vi "load_I_T_from_file.vi"() -> ()   [LabVIEW 2016]
uses:
  <vilib>/Utility/file.llb/Read Delimited Spreadsheet (DBL).vi
panel:
  out "Inputs Shuffled":dbl[][](array[numeric])
  out "Targets Shuffled":dbl[][](array[numeric])
  in  "Proceed to Input Data":bool
  in  "# Nodes Per Stage":dbl[](array[numeric])
  in  "# Hidden Layers":dbl
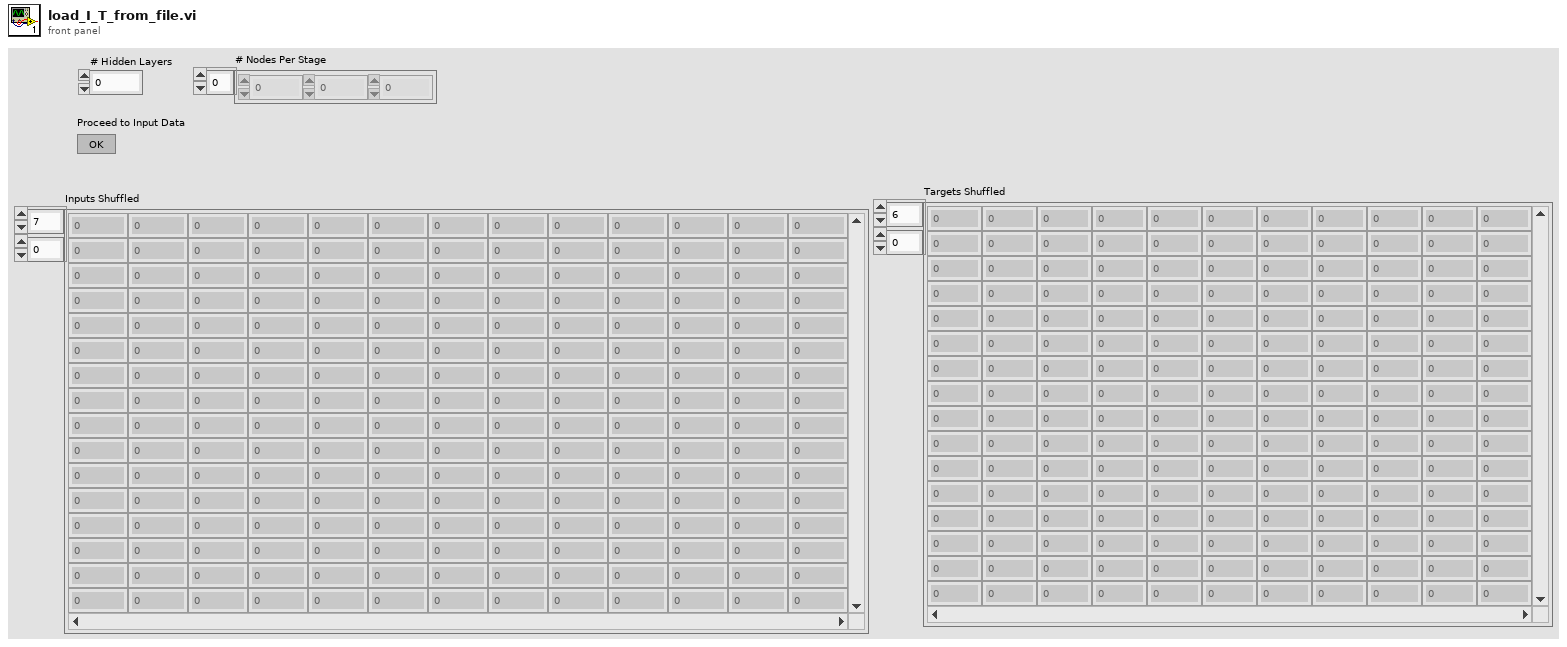
[diagram p1: front panel]
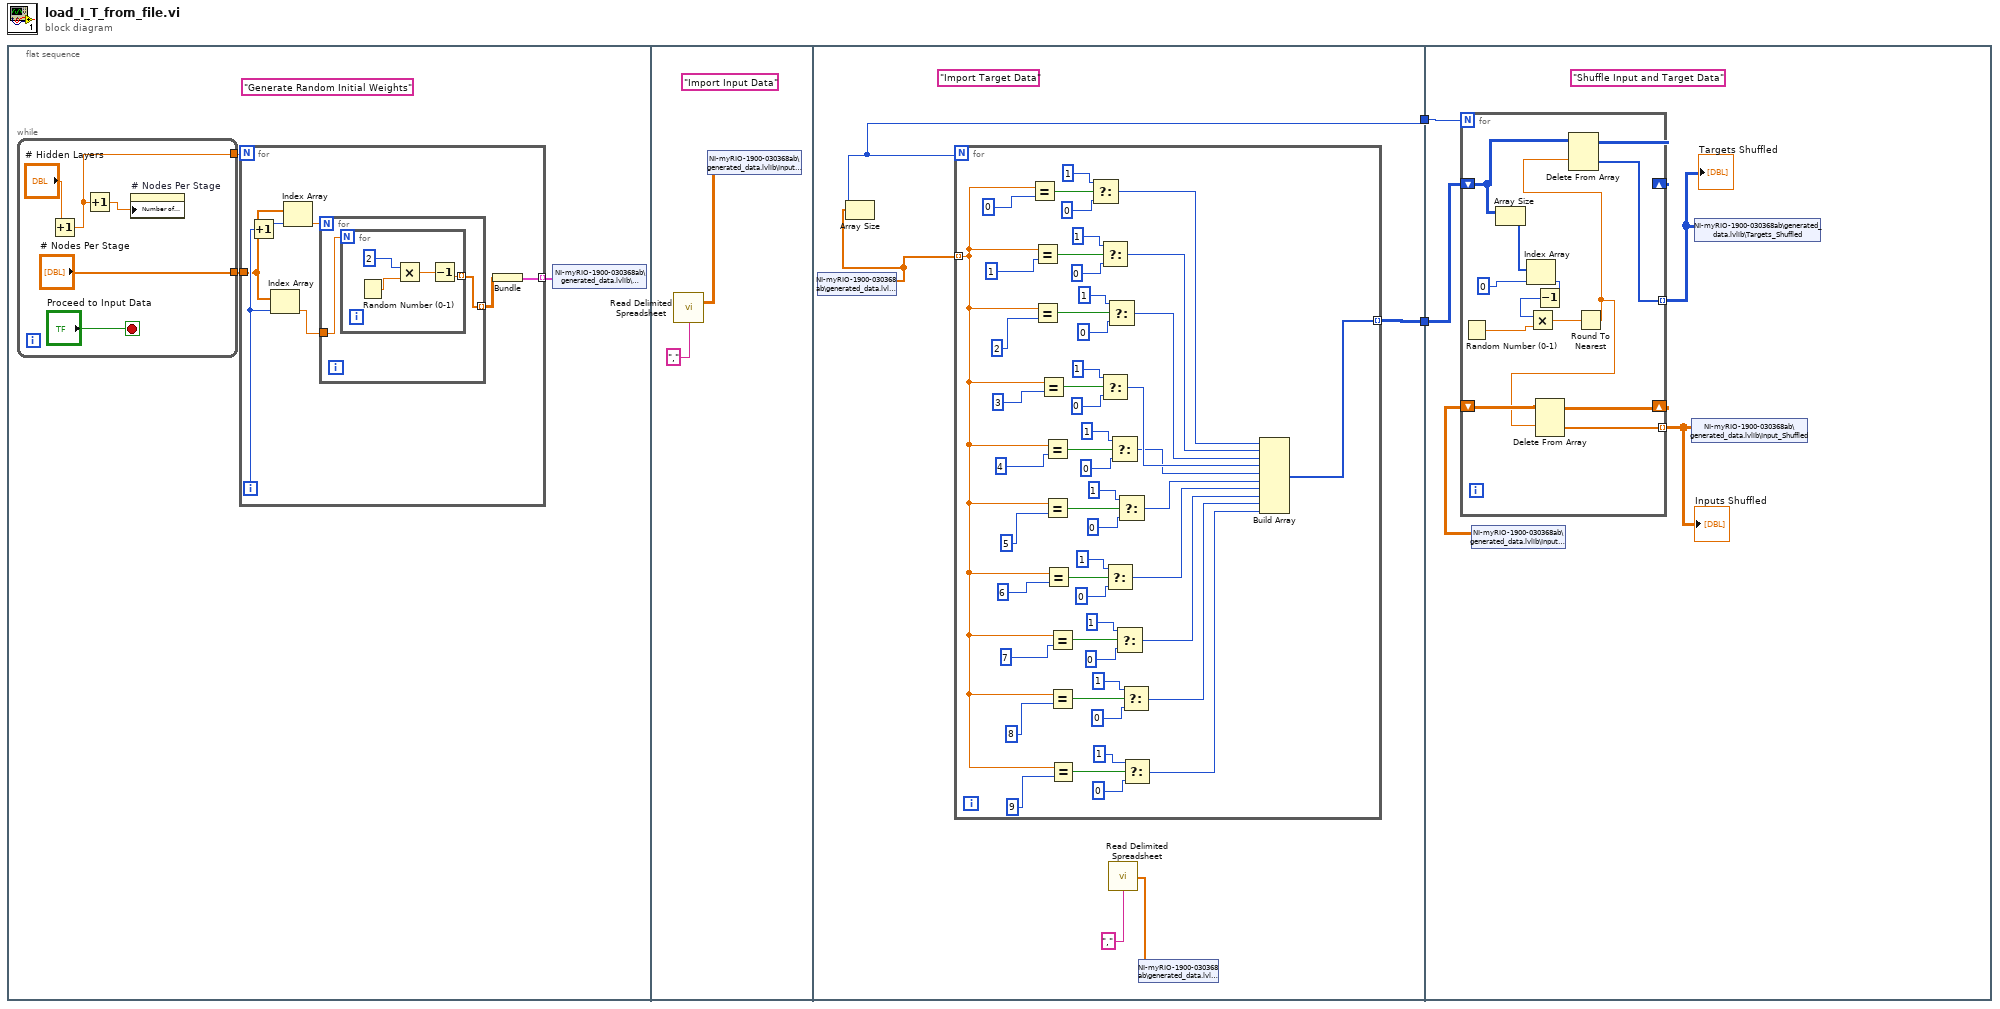
[diagram p0: block diagram]
diagram:
  n1 = flat-sequence {
    tunnel: [w28] -> w2
    tunnel: [w27] -> w1
    tunnel: w2 -> [w87]
    tunnel: w1 -> [w83]
    frame #0 {
      (unwired) "Generate Random Initial Weights"
      n2 = while {
        tunnel: [w8] -> w4
        tunnel: ["# Nodes Per Stage"] -> w3
        stop <- "Proceed to Input Data" stop-if-true
        n3 = Increment(x="# Hidden Layers") -> (x+1=w8:dbl)
        n4 = Increment(x=w8) -> (x+1=w6:dbl)
        n5 = property on="# Nodes Per Stage" class="Arr (strict)"("Number of Columns"=w6) -> ()  [unwired: 2 in, 2 out]
      }
      n6 = for {
        N: w4 -> [_]
        tunnel: [w17] -> w5 mode=indexing
        tunnel: w3 -> [w14]
        i -> [w16]
        n7 = Increment(x=w16) -> (x+1=w15:i32)
        n8 = Index Array(array=w14, index=w16) -> (element=w12:dbl)
        n9 = Index Array(array=w14, index=w15) -> (element=w13:dbl)
        n10 = for {
          N: w13 -> [_]
          tunnel: [w19] -> w11 mode=indexing
          tunnel: w12 -> [w18]
          n11 = for {
            N: w18 -> [_]
            tunnel: [w23] -> w19 mode=indexing
            n12 = Random Number (0-1)() -> (number: 0 to 1=w21:dbl)
            n13 = Multiply(x=2, y=w21) -> (x*y=w20:dbl)
            n14 = Decrement(x=w20) -> (x-1=w23:dbl)
          }
        }
        n15 = Bundle(w11) -> (w17:cluster{dbl[][]})  [unwired: 1 in]
      }
      n16 = shared-variable "NI-myRIO-1900-030368ab\\generated_data.lvlib\\Weights_1"(w5) -> ()  [unwired: 1 in, 1 out]
    }
    frame #1 {
      (unwired) "Import Input Data"
      n17 = call-poly <vilib>:"Read Delimited Spreadsheet.vi"("delimiter (\\t)"=",") -> ("all rows"=w24:dbl[][])  [unwired: 9 in, 5 out]
      n18 = shared-variable "NI-myRIO-1900-030368ab\\generated_data.lvlib\\Input Data"(w24) -> ()  [unwired: 1 in, 1 out]
    }
    frame #2 {
      (unwired) "Import Target Data"
      n19 = shared-variable "NI-myRIO-1900-030368ab\\generated_data.lvlib\\Targets"() -> (w26:dbl[])  [unwired: 1 in, 1 out]
      n20 = Array Size(array=w26) -> (size(s)=w27:i32)
      n21 = for {
        N: w27 -> [_]
        tunnel: w26 -> [w39] mode=indexing
        tunnel: [w67] -> w28 mode=indexing
        n22 = Equal?(x=w39, y=0) -> (x = y?=w79:bool)
        n23 = Equal?(x=w39, y=1) -> (x = y?=w71:bool)
        n24 = Equal?(x=w39, y=2) -> (x = y?=w72:bool)
        n25 = Equal?(x=w39, y=3) -> (x = y?=w63:bool)
        n26 = Equal?(x=w39, y=4) -> (x = y?=w55:bool)
        n27 = Equal?(x=w39, y=5) -> (x = y?=w56:bool)
        n28 = Equal?(x=w39, y=6) -> (x = y?=w51:bool)
        n29 = Equal?(x=w39, y=7) -> (x = y?=w43:bool)
        n30 = Equal?(x=w39, y=8) -> (x = y?=w44:bool)
        n31 = Equal?(x=w39, y=9) -> (x = y?=w40:bool)
        n32 = Select(t=1, s=w79, f=0) -> (s? t:f=w70:i32)
        n33 = Select(t=1, s=w71, f=0) -> (s? t:f=w69:i32)
        n34 = Select(t=1, s=w63, f=0) -> (s? t:f=w38:i32)
        n35 = Select(t=1, s=w51, f=0) -> (s? t:f=w35:i32)
        n36 = Select(t=1, s=w72, f=0) -> (s? t:f=w68:i32)
        n37 = Select(t=1, s=w55, f=0) -> (s? t:f=w37:i32)
        n38 = Select(t=1, s=w43, f=0) -> (s? t:f=w34:i32)
        n39 = Select(t=1, s=w56, f=0) -> (s? t:f=w36:i32)
        n40 = Select(t=1, s=w44, f=0) -> (s? t:f=w33:i32)
        n41 = Select(t=1, s=w40, f=0) -> (s? t:f=w32:i32)
        n42 = Build Array(w70, w69, w68, w38, w37, w36, w35, w34, w33, w32) -> (w67:i32[])
      }
      n43 = call-poly <vilib>:"Read Delimited Spreadsheet.vi"("delimiter (\\t)"=",") -> ("first row"=w30:dbl[])  [unwired: 9 in, 5 out]
      n44 = shared-variable "NI-myRIO-1900-030368ab\\generated_data.lvlib\\Targets"(w30) -> ()  [unwired: 1 in, 1 out]
    }
    frame #3 {
      (unwired) "Shuffle Input and Target Data"
      n45 = shared-variable "NI-myRIO-1900-030368ab\\generated_data.lvlib\\Input Data"() -> (w84:dbl[][])  [unwired: 1 in, 1 out]
      n46 = for {
        N: w83 -> [_]
        shift-right: [w100] -> _
        shift-left: w87 -> [w99]
        tunnel: [w90] -> w86 mode=indexing
        shift-right: [w92] -> _
        shift-left: w84 -> [w93]
        tunnel: [w89] -> w85 mode=indexing
        n47 = Random Number (0-1)() -> (number: 0 to 1=w98:dbl)
        n48 = Array Size(array=w99) -> (size(s)=w96:i32[])
        n49 = Index Array(array=w96, index=0) -> (element=w95:i32)
        n50 = Decrement(x=w95) -> (x-1=w88:i32)
        n51 = Multiply(x=w88, y=w98) -> (x*y=w97:dbl)
        n52 = Round To Nearest(number=w97) -> (nearest integer value=w91:dbl)
        n53 = Delete From Array(array=w93, index (row)=w91) -> (deleted portion=w89:dbl[], array with subset deleted=w92:dbl[][])  [unwired: 2 in]
        n54 = Delete From Array(array=w99, index (row)=w91) -> (deleted portion=w90:i32[], array with subset deleted=w100:i32[][])  [unwired: 2 in]
      }
      "Targets Shuffled" <- w86
      "Inputs Shuffled" <- w85
      n55 = shared-variable "NI-myRIO-1900-030368ab\\generated_data.lvlib\\Input_Shuffled"(w85) -> ()  [unwired: 1 in, 1 out]
      n56 = shared-variable "NI-myRIO-1900-030368ab\\generated_data.lvlib\\Targets_Shuffled"(w86) -> ()  [unwired: 1 in, 1 out]
    }
  }
